vi "Add External Forces.vi"(7 "Gravity":u16, 9 "Angle":dbl[unit], 11 "Mass Distance":dbl[unit]) -> (3 "Torque":dbl[unit])   [LabVIEW 2020]
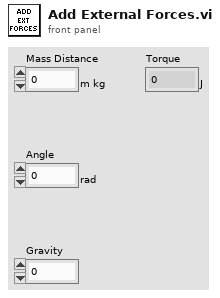
[diagram p1: front panel]
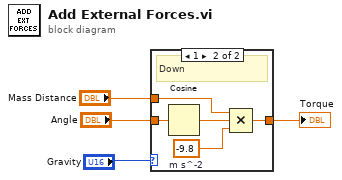
[diagram p0: block diagram]
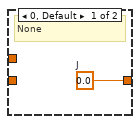
[diagram p2: hidden frame]
diagram:
  n1 = case shown="1" "Gravity" {
    tunnel: "Mass Distance" -> [_ w9]
    tunnel: [w5 w8] -> w2
    tunnel: "Angle" -> [_ w6]
    frame 0, Default {
      w5 = dbl[unit] 0.0  # J
      # "None"
    }
    frame 1 {
      w7 = dbl[unit] -9.8  # m s^-2
      # "Down"
      n2 = Cosine(x=w6) -> (cos(x)=w10:dbl)
      n3 = Compound Arithmetic op=MULTIPLY(w9, w10, w7) -> (w8:dbl[unit])
    }
  }
  "Torque" <- w2
